vi "GFITS_IncNumber.vi"(8 "error in (no error)":errorcluster, 11 "Database RefNum":T1) -> (0 "error out":errorcluster)   [LabVIEW 2016]
uses:
  DBSHAND/private/vis/DatabaseHand_RefNum.ctl
  DBSHAND/private/vis/DatabaseHand_Element_Get(bool).vi
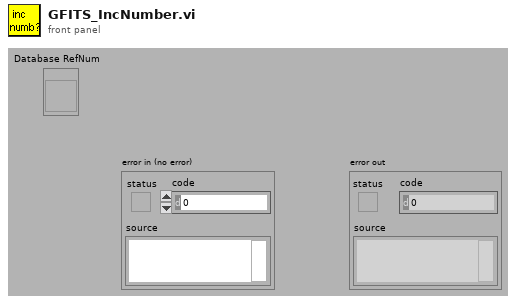
[diagram p1: front panel]
types:
  T1 = typedef "DatabaseHand_RefNum.ctl" = refnum<vi>
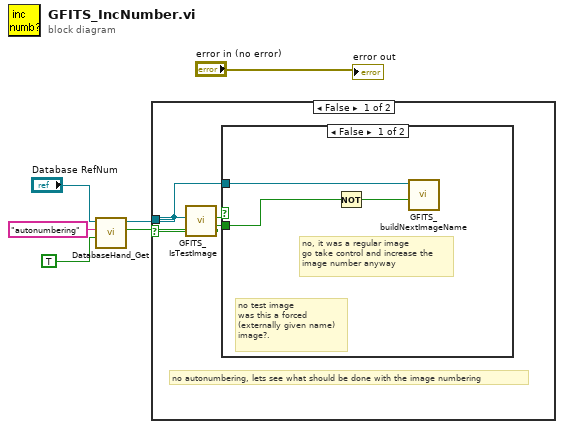
[diagram p0: block diagram]
diagram:
  n1 = call-poly "DatabaseHand_Get.vi"("default value"=TRUE, "name"="autonumbering", "Database RefNum in"="Database RefNum") -> ("value"=w3:bool, "Database RefNum out"=w2:T1)  [unwired: 2 in, 5 out]
  n2 = case shown="False" w3 {
    tunnel: w2 -> [w8 _]
    frame False {
      # "no autonumbering, lets see what should be done with the image numbering"
      n3 = call "GFITS_IsTestImage.vi"("Database RefNum in"=w8) -> ("forcedfits?"=w7:bool, "testonly"=w9:bool)  [unwired: 9 out]
      n4 = case shown="False" w9 {
        tunnel: w8 -> [w12 _]
        tunnel: w7 -> [w11 _]
        frame False {
          # "no, it was a regular image\ngo take control and increase the\nimage number anyway"
          # "no test image\nwas this a forced\n(externally given name)\nimage?."
          n5 = Not(x=w11) -> (.not. x?=w10:bool)
          n6 = call "GFITS_buildNextImageName.vi"("incnumber"=w10, "Database RefNum"=w12) -> ()  [unwired: 1 in, 7 out]
        }
        frame True {
          # "is this a testimage (testmode on fits server)\nif so, do nothing"
        }
      }
    }
    frame True {
      # "autonumbering is the usual way of numbering, where the control\nis taken over the Logic subprocesses to increase the image number"
    }
  }
  "error out" <- "error in (no error)"
